vi "Chirp_MeasurementV3.vi"(8 "error in (no error) 2":errorcluster, 11 "ChirpV2 in 2":refnum<class "ChirpV2.lvclass">) -> (0 "error out 2":errorcluster, 2 "data 3":dynamicdata(graph) caption="data", 3 "ChirpV2 out 2":refnum<class "ChirpV2.lvclass">)   [LabVIEW 2014, in "ChirpV2.lvclass"]
uses:
  ChirpV2.lvclass
  <vilib>/Analysis/4window.llb/Cosine Tapered Window (DBL).vi
  <vilib>/measure/NI_MABase.lvlib
  <vilib>/addons/_NISVFA/_Generation/SoundVib_Generation.lvlib
  <vilib>/Analysis/NI_AALPro.lvlib
panel:
  out "Duration":dbl
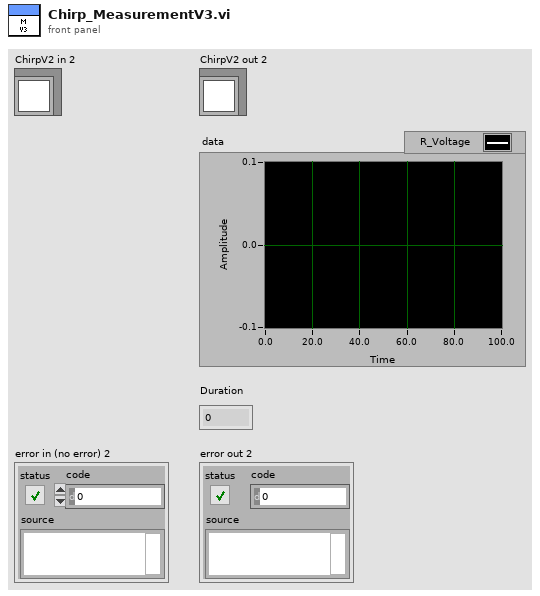
[diagram p1: front panel]
types:
  T1 = cluster{"start frequency [Hz]":dbl, "stop frequency [Hz]":dbl}
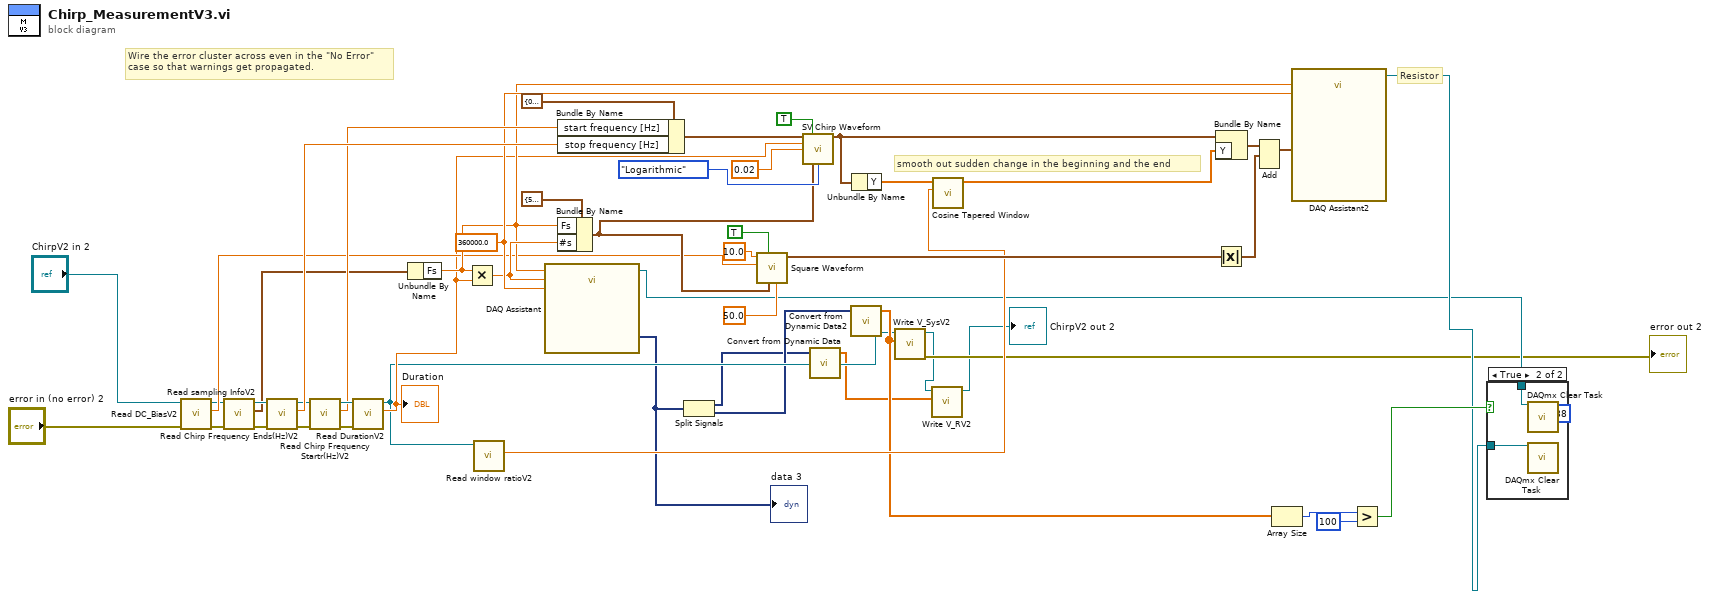
[diagram p0: block diagram]
diagram:
  (unwired) 200088 ("specific error code to clear (0: all)")
  w34 = 360000.0 ("timeout (s)")
  # "smooth out sudden change in the beginning and the end"
  # "Resistor"
  # "Wire the error cluster across even in the \"No Error\"\ncase so that warnings get propagated."
  n1 = call-dynamic "Read DC_BiasV2.vi"("error in (no error)"="error in (no error) 2", "ChirpV2 in"="ChirpV2 in 2") -> ("error out"=w22:errorcluster, "DC_Bias"=w23:dbl, "ChirpV2 out"=w21:refnum<class "ChirpV2.lvclass">)  [unwired: 7 in]
  n2 = call-dynamic "Read sampling InfoV2.vi"("error in (no error)"=w22, "ChirpV2 in"=w21) -> ("error out"=w42:errorcluster, "sampling Info"=w24:cluster{"Fs":dbl}, "ChirpV2 out"=w37:refnum<class "ChirpV2.lvclass">)  [unwired: 7 in]
  n3 = call-dynamic "Read Chirp Frequency Ends(Hz)V2.vi"("error in (no error)"=w42, "ChirpV2 in"=w37) -> ("error out"=w43:errorcluster, "Chirp Frequency Ends(Hz)"=w41:dbl, "ChirpV2 out"=w38:refnum<class "ChirpV2.lvclass">)  [unwired: 7 in]
  n4 = call-dynamic "Read Chirp Frequency Startr(Hz)V2.vi"("error in (no error)"=w43, "ChirpV2 in"=w38) -> ("error out"=w46:errorcluster, "Chirp Frequency Startr(Hz)"=w40:dbl, "ChirpV2 out"=w45:refnum<class "ChirpV2.lvclass">)  [unwired: 7 in]
  n5 = call-dynamic "Read DurationV2.vi"("error in (no error)"=w46, "ChirpV2 in"=w45) -> ("Duration"=w16:dbl, "ChirpV2 out"=w7:refnum<class "ChirpV2.lvclass">)  [unwired: 7 in, 1 out]
  "Duration" <- w16
  n6 = Unbundle By Name(w24) -> ("Fs"=w32:dbl)
  n7 = Multiply(x=w32, y=w16) -> (x*y=w33:dbl)
  n8 = call-dynamic "Read window ratioV2.vi"("ChirpV2 in"=w7) -> ("window ratio"=w15:dbl)  [unwired: 8 in, 2 out]
  n9 = call "DAQ Assistant"("rate"=w32, "number of samples"=w33, "timeout (s)"=w34) -> ("task out"=w10:refnum<k21>, "data"=w6:dynamicdata)  [unwired: 14 in, 1 out]
  "data 3" <- w6
  n10 = Bundle By Name(cluster=T1 {"start frequency [Hz]"=0.01, "stop frequency [Hz]"=10.0} ("frequency range"), "start frequency [Hz]"=w40, "stop frequency [Hz]"=w41) -> (w44:T1)
  n11 = Bundle By Name(cluster=cluster{"Fs":dbl, "#s":u32} {"Fs"=51200.0, "#s"=1024} ("sampling info"), "Fs"=w32, "#s"=w33) -> (w26:cluster{"Fs":dbl, "#s":u32})
  n12 = Split Signals(w6) -> (w4:dynamicdata, w5:dynamicdata)  [unwired: 2 in]
  n13 = call <vilib>:"Square Waveform.vi"("duty cycle (%)"=50.0, "sampling info"=w26, "reset signal"=TRUE, "amplitude"=w23, "frequency"=10.0) -> ("signal out"=w19:waveform(dbl))  [unwired: 5 in, 1 out]
  n14 = call <vilib>:"SV Chirp Waveform.vi"("frequency range"=w44, "reset signal (F)"=TRUE, "chirp duration [s]"=w16, "amplitude"=0.02, "sampling info"=w26, "frequency spacing"=enum16{"Linear", "Logarithmic"}."Logarithmic") -> ("chirp signal"=w47:waveform(dbl))  [unwired: 7 in, 2 out]
  n15 = call "Convert from Dynamic Data"("Dynamic Data Type"=w4) -> ("Array"=w1:dbl[])  [unwired: 3 in]
  n16 = call "Convert from Dynamic Data2"("Dynamic Data Type"=w5) -> ("Array"=w9:dbl[])  [unwired: 3 in]
  n17 = Unbundle By Name(w47) -> ("Y"=w48:dbl[])
  n18 = call-dynamic "Write V_SysV2.vi"("V_Sys"=w9, "ChirpV2 in"=w7) -> ("error out"=→"error out 2":errorcluster, "ChirpV2 out"=w3:refnum<class "ChirpV2.lvclass">)  [unwired: 8 in]
  n19 = call-dynamic "Write V_RV2.vi"("V_R"=w1, "ChirpV2 in"=w3) -> ("ChirpV2 out"=→"ChirpV2 out 2":refnum<class "ChirpV2.lvclass">)  [unwired: 8 in, 1 out]
  n20 = call-poly <vilib>:"Cosine Tapered Window.vi"("ratio"=w15, "X"=w48) -> ("Windowed X"=w49:dbl[])  [unwired: 8 in, 1 out]
  n21 = Bundle By Name(cluster=w47, "Y"=w49) -> (w50:waveform(dbl))
  n22 = Absolute Value(x=w19) -> (abs(x)=w28:waveform(dbl))
  n23 = Add(1:w28, 2:w50) -> (0:w29:waveform(dbl))  [unwired: 1 in, 1 out]
  n24 = Array Size(array=w9) -> (size(s)=w14:i32)
  n25 = call "DAQ Assistant2"("data"=w29, "rate"=w32, "timeout (s)"=w34) -> ("task out"=w11:refnum<k21>)  [unwired: 14 in, 2 out]
  n26 = Greater?(x=w14, y=100) -> (0:w13:bool)
  n27 = case shown="True" w13 {
    tunnel: w11 -> [_ w52]
    tunnel: w10 -> [_ w51]
    frame False {
    }
    frame True {
      n28 = call <vilib>:"DAQmx Clear Task.vi"("task in"=w51) -> ()  [unwired: 14 in, 1 out]
      n29 = call <vilib>:"DAQmx Clear Task.vi"("task in"=w52) -> ()  [unwired: 14 in, 1 out]
    }
  }
